vi "sithermalchecksum.vi"(0 "Array":dbl[](array[numeric])) -> (1 "Lower Checksum":u8, 2 "Upper Checksum":u8)   [LabVIEW 2011]
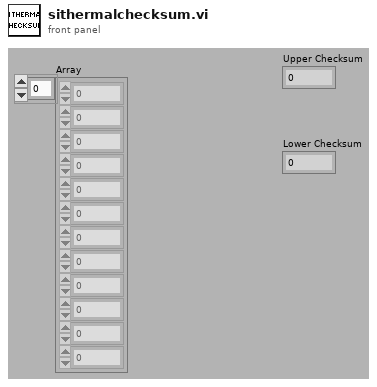
[diagram p1: front panel]
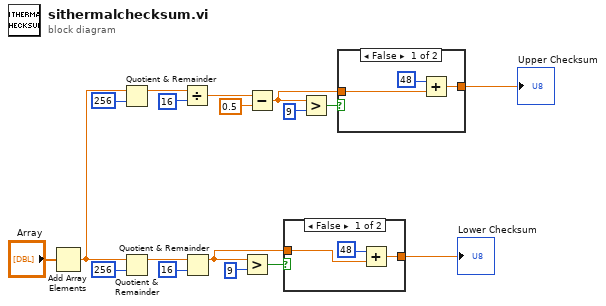
[diagram p0: block diagram]
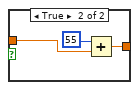
[diagram p2: hidden frame]
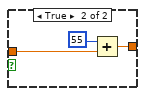
[diagram p3: hidden frame]
diagram:
  n1 = Add Array Elements(numeric array="Array") -> (sum=w5:dbl)
  n2 = Quotient & Remainder(x=w5, y=u16 256) -> (x-y*floor(x/y)=w16:dbl)  [unwired: 1 out]
  n3 = Quotient & Remainder(x=w5, y=u16 256) -> (x-y*floor(x/y)=w7:dbl)  [unwired: 1 out]
  n4 = Divide(x=w16, y=u16 16) -> (x/y=w14:dbl)
  n5 = Quotient & Remainder(x=w7, y=u16 16) -> (x-y*floor(x/y)=w1:dbl)  [unwired: 1 out]
  n6 = Greater?(x=w1, y=u8 9) -> (0:w3:bool)
  n7 = Subtract(x=w14, y=0.5) -> (x-y=w9:dbl)
  n8 = case shown="False" w3 {
    tunnel: w1 -> [w19 w23]
    tunnel: [w20 w22] -> w4
    frame False {
      n9 = Add(x=48, y=w19) -> (x+y=w20:dbl)
    }
    frame True {
      n10 = Add(x=55, y=w23) -> (x+y=w22:dbl)
    }
  }
  "Lower Checksum" <- w4
  n11 = Greater?(x=w9, y=u8 9) -> (0:w11:bool)
  n12 = case shown="False" w11 {
    tunnel: w9 -> [w25 w29]
    tunnel: [w26 w28] -> w12
    frame False {
      n13 = Add(x=48, y=w25) -> (x+y=w26:dbl)
    }
    frame True {
      n14 = Add(x=55, y=w29) -> (x+y=w28:dbl)
    }
  }
  "Upper Checksum" <- w12
